vi "GetCustomDevicePageVIs.vi"(8 "error in (no error)":errorcluster, 11 "custom device reference in":refnum<k39>) -> (0 "error out":errorcluster, 2 "page VIs":T1(array[cluster]), 3 "custom device reference out":refnum<k39>)   [LabVIEW 2027, in "VeriStandTestUtilities.lvlib"]
uses:
  VeriStandTestUtilities.lvlib
  C:/NetCoreDLL/NationalInstruments.VeriStand.XMLReader.dll
  NetCoreDLL/NationalInstruments.VeriStand.XMLReader.dll
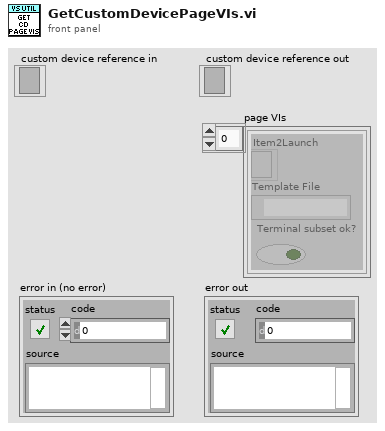
[diagram p1: front panel]
types:
  T1 = cluster{"Item2Launch":refnum<k39>, "Template File":path, "Terminal subset ok?":bool}[]
  T2 = cluster{"Item2Launch":refnum<k39>, "Template File":path, bool}
  T3 = cluster{"Item2Launch":refnum<k39>, "Template File":path, bool}[]
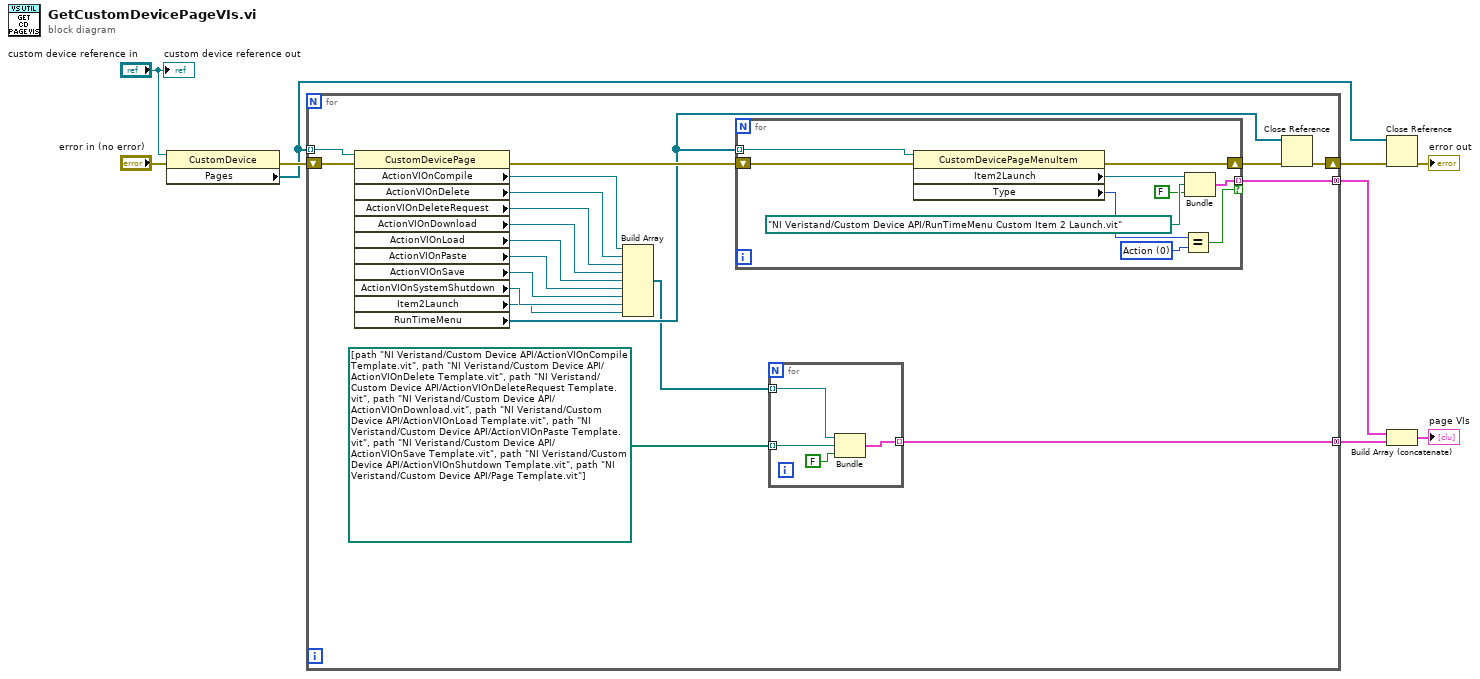
[diagram p0: block diagram]
diagram:
  n1 = property class="CustomDevice"(reference="custom device reference in", error in="error in (no error)") -> (error out=w8:errorcluster, "Pages"=w3:refnum<k39>[])  [unwired: 1 out]
  n2 = for {
    tunnel: w3 -> [w28] mode=indexing
    tunnel: [w27] -> w2 mode=concatenating
    shift-right: [w23] -> w6
    shift-left: w8 -> [w24]
    tunnel: [w10] -> w1 mode=concatenating
    n3 = property class="CustomDevicePage"(reference=w28, error in=w24) -> (error out=w25:errorcluster, "ActionVIOnCompile"=w21:refnum<k39>, "ActionVIOnDelete"=w20:refnum<k39>, "ActionVIOnDeleteRequest"=w19:refnum<k39>, "ActionVIOnDownload"=w18:refnum<k39>, "ActionVIOnLoad"=w17:refnum<k39>, "ActionVIOnPaste"=w16:refnum<k39>, "ActionVIOnSave"=w15:refnum<k39>, "ActionVIOnSystemShutdown"=w14:refnum<k39>, "Item2Launch"=w13:refnum<k39>, "RunTimeMenu"=w22:refnum<k39>[])  [unwired: 1 out]
    n4 = Build Array(w21, w20, w19, w18, w17, w16, w15, w14, w13) -> (w12:refnum<k39>[])
    n5 = for {
      tunnel: w22 -> [w38] mode=indexing
      tunnel: [w33] -> w27 mode=indexing if=w35
      shift-right: [w31] -> w26
      shift-left: w25 -> [w30]
      w34 = 0 items=["Action", "VI", "Separator", "Custom"] ("Type")
      n6 = property class="CustomDevicePageMenuItem"(reference=w38, error in=w30) -> (error out=w31:errorcluster, "Item2Launch"=w37:refnum<k39>, "Type"=w36:i32)  [unwired: 1 out]
      n7 = Equal?(x=w36, y=w34) -> (x = y?=w35:bool)
      n8 = Bundle("Item2Launch"=w37, "Template File"=path "NI Veristand/Custom Device API/RunTimeMenu Custom Item 2 Launch.vit", FALSE) -> (w33:T2)  [unwired: 1 in]
    }
    n9 = for {
      tunnel: w12 -> [w42] mode=indexing
      tunnel: path[] [path "NI Veristand/Custom Device API/ActionVIOnCompile Template.vit", path "NI Veristand/Custom Device API/ActionVIOnDelete Template.vit", path "NI Veristand/Custom Device API/ActionVIOnDeleteRequest Template.vit", path "NI Veristand/Custom Device API/ActionVIOnDownload.vit", path "NI Veristand/Custom Device API/ActionVIOnLoad Template.vit", path "NI Veristand/Custom Device API/ActionVIOnPaste Template.vit", path "NI Veristand/Custom Device API/ActionVIOnSave Template.vit", path "NI Veristand/Custom Device API/ActionVIOnShutdown Template.vit", path "NI Veristand/Custom Device API/Page Template.vit"] -> [w41] mode=indexing
      tunnel: [w40] -> w10 mode=indexing
      n10 = Bundle("Item2Launch"=w42, w41, FALSE) -> (w40:cluster{"Item2Launch":refnum<k39>, path, bool})  [unwired: 1 in]
    }
    n11 = Close Reference(reference=w22, error in (no error)=w26) -> (error out=w23:errorcluster)
  }
  n12 = Close Reference(reference=w3, error in (no error)=w6) -> (error out=→"error out":errorcluster)
  n13 = Build Array (concatenate)(w2, w1) -> (→"page VIs":T3)
  "custom device reference out" <- "custom device reference in"
